vi "10kv set steerer.vi"(8 "error in":errorcluster, 10 "Steerer Control IN":dbl(knob) scale=-10.0..10.0 scale format="%#_4g") -> (0 "error out":errorcluster, 1 "- Steerer":dbl, 2 "+ Steerer":dbl)   [LabVIEW 2009]
doc: "This takes an input for a steerer and converts it into \nits positive and negaitve components. This is set \nfor a 10kv supplies"
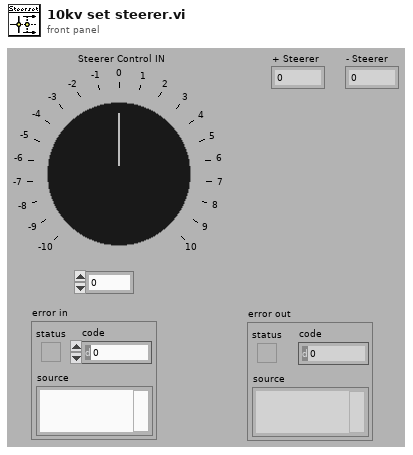
[diagram p1: front panel]
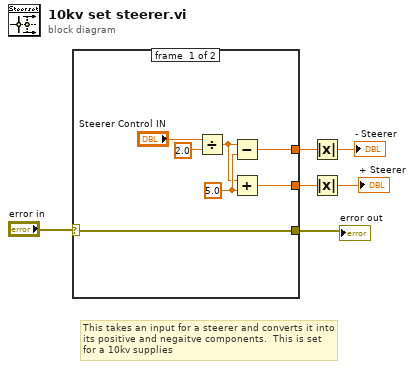
[diagram p0: block diagram]
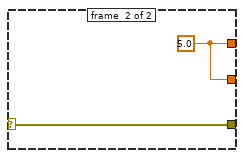
[diagram p2: hidden frame]
diagram:
  # "This takes an input for a steerer and converts it into \nits positive and negaitve components.  This is set \nfor a 10kv supplies"
  n1 = case shown="No Error" "error in" {
    selector: "error in" -> [w7 w14]
    tunnel: [w13 w15] -> w4
    tunnel: [w12 w15] -> w2
    tunnel: [w7 w14] -> w5
    frame #0 {
      w11 = 5.0 ("y")
      n2 = Divide(x="Steerer Control IN", y=2.0) -> (x/y=w10:dbl)
      n3 = Subtract(x=w10, y=w11) -> (x-y=w13:dbl)
      n4 = Add(x=w10, y=w11) -> (x+y=w12:dbl)
    }
    frame #1 {
      w15 = 5.0
    }
  }
  "error out" <- w5
  n5 = Absolute Value(x=w4) -> (abs(x)=→"- Steerer":dbl)
  n6 = Absolute Value(x=w2) -> (abs(x)=→"+ Steerer":dbl)
